vi "Convert2Voltage.vi"(11 "SRP ADC String":string="00000000") -> (3 "Voltage":dbl)   [LabVIEW 2011]
doc: "This VI converts the input SRP ADC string to a voltage.\n\nInputs:\n1.SRP ADC String: This is 8 bit, hexadecimal string provided by the SRP when doing a measuremnt.\n\nOutputs:\n1.Voltage: This is the voltage read."
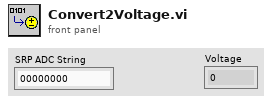
[diagram p1: front panel]
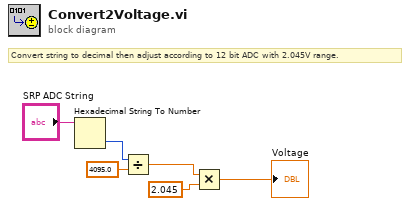
[diagram p0: block diagram]
diagram:
  # "Convert string to decimal then adjust according to 12 bit ADC with 2.045V range."
  n1 = Hexadecimal String To Number(string="SRP ADC String") -> (number=w5:u32)  [unwired: 2 in, 1 out]
  n2 = Divide(x=w5, y=4095.0) -> (x/y=w2:dbl)
  n3 = Multiply(x=w2, y=2.045) -> (x*y=→"Voltage":dbl)
